vi "Plot Update Cursor 1D Table.vi"(6 "Cursor XYZ":T1, 8 "Data 1D Table":cluster{"X":sgl[], "Y":sgl[]}, 11 "Table Ref":refnum<vi>) -> ()   [LabVIEW 2016]
uses:
  <vilib>/addons/Software Calibration Management/xSCM/Controls/TLU2D.ctl
  <vilib>/Utility/miscctls.llb/LVRowAndColumnTypeDef.ctl
  <vilib>/addons/Software Calibration Management/xSCM/SCM-API.lvlib
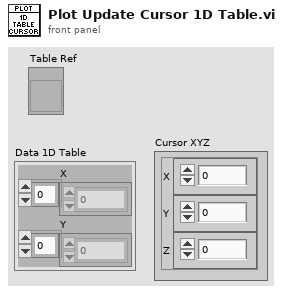
[diagram p1: front panel]
types:
  T1 = typedef "SCM-API.lvlib/TLU2D.ctl" = cluster{"X":sgl, "Y":sgl, "Z":sgl}
  T2 = typedef "LVRowAndColumnTypeDef.ctl" = cluster{"Row":i32, "Column":i32}
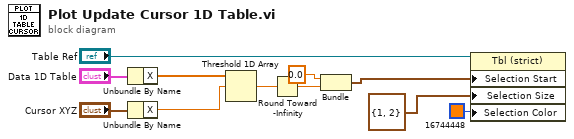
[diagram p0: block diagram]
diagram:
  n1 = Unbundle By Name("Data 1D Table") -> ("X"=w10:sgl[])
  n2 = Unbundle By Name("Cursor XYZ") -> ("X"=w9:sgl)
  n3 = Threshold 1D Array(2:w9, 3:w10) -> (0:w8:sgl)  [unwired: 1 in]
  n4 = Round Toward -Infinity(1:w8) -> (0:w2:sgl)
  n5 = Bundle("floor(x): largest int <= x"=sgl 0.0, w2) -> (w5:cluster{"floor(x): largest int <= x":sgl, sgl})  [unwired: 1 in]
  n6 = property on="Property Node" class="Tbl (strict)"(reference="Table Ref", "Selection Start"=w5, "Selection Size"=T2 {"Row"=1, "Column"=2}, "Selection Color"=u32 16744448) -> ()  [unwired: 1 in, 2 out]
